vi "Send Command.vi"(6 "Command in":T1, 8 "error in":errorcluster, 10 "Value":dbl, 11 "Kronos in":refnum<class "Kronos.lvclass">) -> (0 "error out":errorcluster, 3 "Kronos out":refnum<class "Kronos.lvclass">, 4 "Command out":T1)   [LabVIEW 2018, in "Kronos.lvlib" / "Kronos.lvclass"]
uses:
  Kronos.lvclass
  PPLs/Laser/Parent/Laser.lvlibp/Custom Controls/Command List.ctl
  Kronos.lvclass/Kronos.ctl
  PPLs/Laser/Parent/Laser.lvlibp/Laser.lvclass
  C:/AME Test Engineering/LabVIEW/PPLs/Laser/Parent/Laser.lvlibp/Laser.lvclass
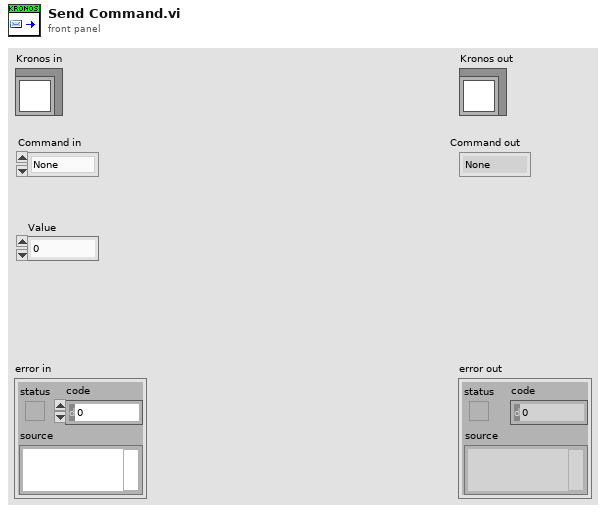
[diagram p1: front panel]
types:
  T1 = typedef "Laser.lvlibp/Laser.lvclass/Command List.ctl" = enum16{"None", "Config?", "Volt?", "ThCase?", "STS?", "Mon?", "Help?", "HB", "Verbose", "Spnt", "Ext", "PRF", "Start", "Stop", "PRF?", "State?", "Status?", "Stat?", "Read HB", "Logon", "Poutmax", "saveconfig", "Reset", "Poutmax?", "PoutCommandMax", "PoutCommandMax?", "FreqMin", "FreqMin?"}
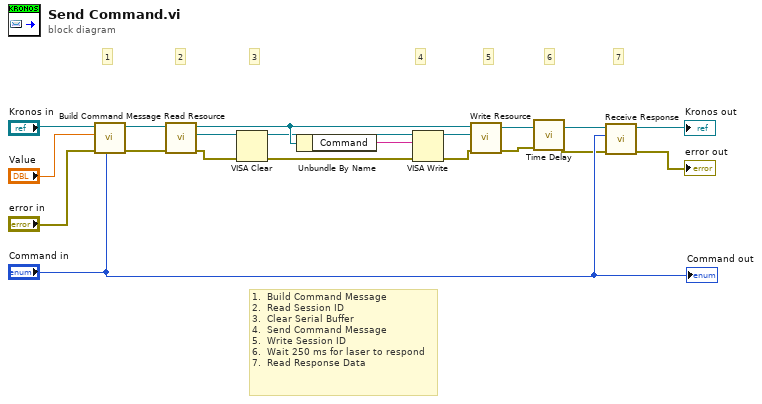
[diagram p0: block diagram]
diagram:
  # "7"
  # "6"
  # "1.  Build Command Message\n2.  Read Session ID\n3.  Clear Serial Buffer\n4.  Send Command Message \n5.  Write Session ID\n6.  Wait 250 ms for laser to respond\n7.  Read Response Data"
  # "5"
  # "4"
  # "3"
  # "2"
  # "1"
  n1 = call "Build Command Message.vi"("Command"="Command in", "error in"="error in", "Parameter"="Value", "Kronos in"="Kronos in") -> ("error out"=w16:errorcluster, "Kronos out"=w15:refnum<class "Kronos.lvclass">)  [unwired: 6 in]
  n2 = call "Read Resource.vi"("error in (no error)"=w16, "Laser in"=w15) -> ("error out"=w8:errorcluster, "Resource"=w10:refnum<visa-resource-name>, "Laser out"=w11:refnum<class "Kronos.lvclass">)  [unwired: 7 in]
  n3 = VISA Clear(VISA resource name=w10, error in (no error)=w8) -> (VISA resource name out=w9:refnum<visa-resource-name>, error out=w7:errorcluster)
  n4 = Unbundle By Name(w11) -> ("Command"=w13:string)
  n5 = VISA Write(VISA resource name=w9, write buffer=w13, error in (no error)=w7) -> (VISA resource name out=w14:refnum<visa-resource-name>, error out=w12:errorcluster)  [unwired: 1 out]
  n6 = call "Write Resource.vi"("error in (no error)"=w12, "Resource"=w14, "Laser in"=w11) -> ("error out"=w4:errorcluster, "Laser out"=w6:refnum<class "Kronos.lvclass">)  [unwired: 7 in]
  n7 = call "Time Delay"("error in (no error)"=w4) -> ("error out"=w1:errorcluster)  [unwired: 10 in]
  n8 = call-dynamic "Receive Response.vi"("error in"=w1, "Command in"="Command in", "Kronos in"=w6) -> ("error out"=→"error out":errorcluster, "Kronos out"=→"Kronos out":refnum<class "Kronos.lvclass">)  [unwired: 7 in]
  "Command out" <- "Command in"
